vi "Test Step Control.vi"(7 "Step Actions":T1, 8 "error in (no error)":errorcluster, 11 "Test Table":string[][](table)=[[""]]) -> (0 "error out":errorcluster, 1 "Test Running":bool, 2 "Current Test Step Index":i32, 3 "Current Test Step Parameters":string[](array[string]), 5 "Test Table Out":string[][](array[string]))   [LabVIEW 2018]
doc: "Manages the state control of the wash steps.\nAllows setting of the initial steps and then sequencing to the next one"
uses:
  Controls/Step Control Methods ENUM_TEST_TDef.ctl
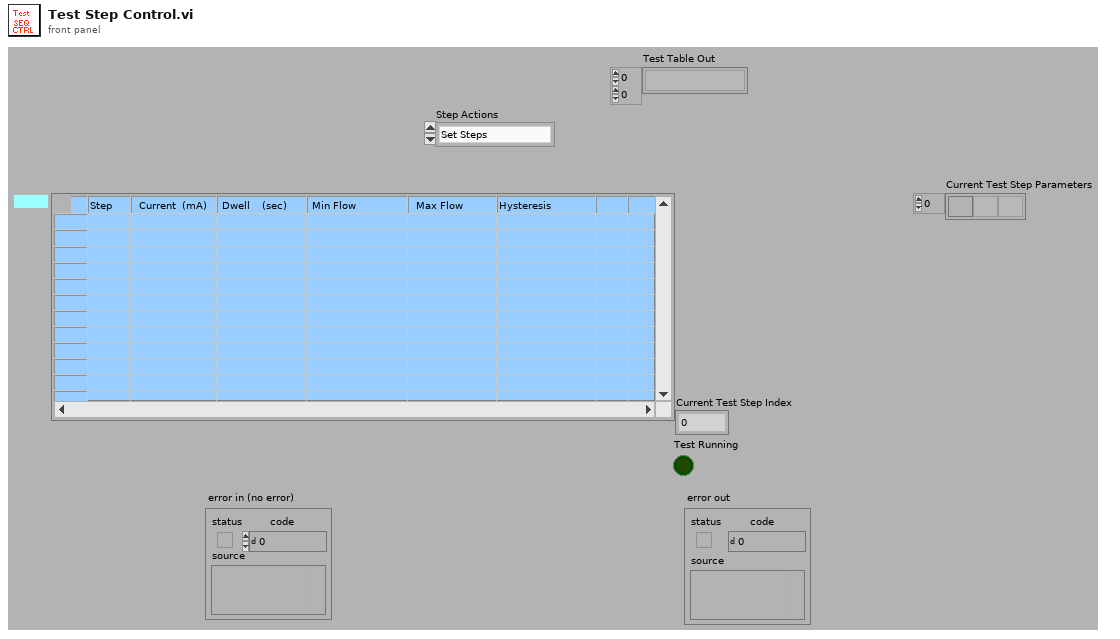
[diagram p1: front panel]
types:
  T1 = typedef "Step Control Methods ENUM_TEST_TDef.ctl" = enum16{"Set Steps", "Get Current", "Goto Previous Step", "Goto Next Step", "Reset"}
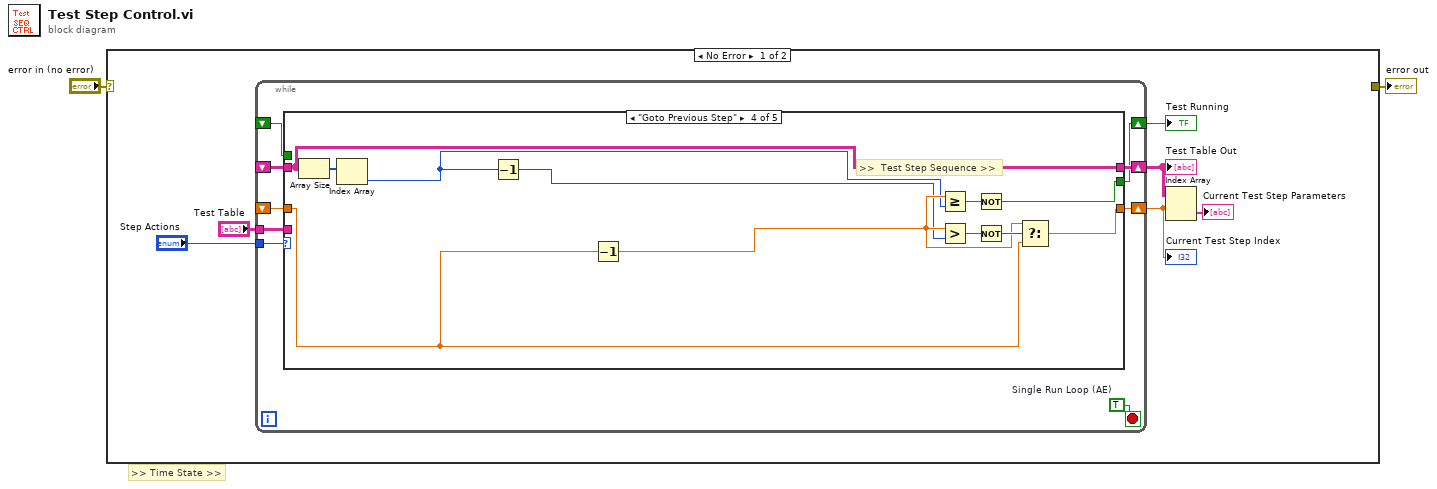
[diagram p0: block diagram]
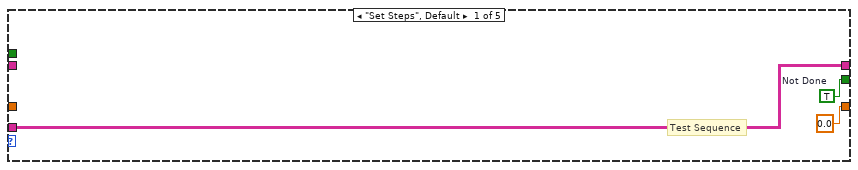
[diagram p2: hidden frame]
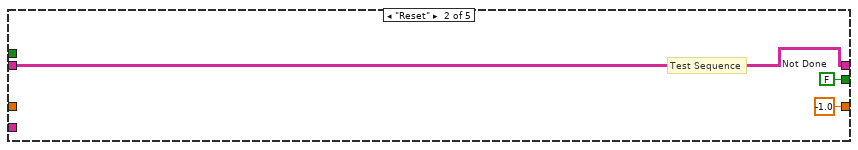
[diagram p3: hidden frame]
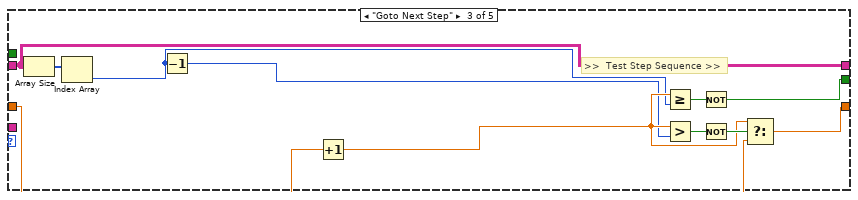
[diagram p4: hidden frame]
diagram:
  # ">> Time State >>"
  n1 = case shown="No Error" "error in (no error)" {
    selector: "error in (no error)" -> [_ w49]
    tunnel: [_ w49] -> w1
    frame No Error {
      n2 = while {
        tunnel: "Step Actions" -> [w16]
        shift-right: [w14] -> w5
        shift-left: _ -> [w13]
        tunnel: "Test Table" -> [w15]
        shift-right: [w12] -> w4
        shift-left: _ -> [w11]
        shift-right: [w10] -> w6
        shift-left: _ -> [w9]
        stop <- w17 stop-if-true
        w17 = TRUE  # Single Run Loop (AE)
        n3 = case shown="\"Goto Previous Step\"" w16 {
          tunnel: w15 -> [w20 _ _ _ _]
          tunnel: [w20 w21 w34 w45 w47] -> w14
          tunnel: w13 -> [_ w21 w34 w45 w47]
          tunnel: [0.0 -1.0 w30 w41 w48] -> w12
          tunnel: w11 -> [_ _ w31 w42 w48]
          tunnel: [w19 w23 w32 w43 w46] -> w10
          tunnel: w9 -> [_ _ _ _ w46]
          frame "Set Steps", Default {
            w19 = TRUE  # Not Done
            # "Test Sequence"
          }
          frame "Reset" {
            w23 = FALSE  # Not Done
            # "Test Sequence"
          }
          frame "Goto Next Step" {
            # ">>  Test Step Sequence >>"
            n4 = Array Size(array=w34) -> (size(s)=w33:i32[])
            n5 = Index Array(array=w33) -> (element=w25:i32)  [unwired: 1 in]
            n6 = Decrement(x=w25) -> (x-1=w24:i32)
            n7 = Increment(x=w31) -> (x+1=w26:dbl)
            n8 = Greater Or Equal?(x=w26, y=w25) -> (x >= y?=w28:bool)
            n9 = Greater?(x=w26, y=w24) -> (0:w27:bool)
            n10 = Not(x=w28) -> (.not. x?=w32:bool)
            n11 = Not(x=w27) -> (.not. x?=w29:bool)
            n12 = Select(t=w26, s=w29, f=w31) -> (s? t:f=w30:dbl)
          }
          frame "Goto Previous Step" {
            # ">>  Test Step Sequence >>"
            n13 = Array Size(array=w45) -> (size(s)=w44:i32[])
            n14 = Index Array(array=w44) -> (element=w36:i32)  [unwired: 1 in]
            n15 = Decrement(x=w36) -> (x-1=w35:i32)
            n16 = Decrement(x=w42) -> (x-1=w37:dbl)
            n17 = Greater Or Equal?(x=w37, y=w36) -> (x >= y?=w39:bool)
            n18 = Greater?(x=w37, y=w35) -> (0:w38:bool)
            n19 = Not(x=w39) -> (.not. x?=w43:bool)
            n20 = Not(x=w38) -> (.not. x?=w40:bool)
            n21 = Select(t=w37, s=w40, f=w42) -> (s? t:f=w41:dbl)
          }
          frame "Get Current" {
          }
        }
      }
      "Current Test Step Index" <- w4
      "Test Running" <- w6
      "Test Table Out" <- w5
      n22 = Index Array(array=w5, index (row)=w4) -> (element=→"Current Test Step Parameters":string[])  [unwired: 1 in]
    }
    frame Error {
    }
  }
  "error out" <- w1
